vi "Pop-up New Error Window.vi"(8 "Error In":errorcluster, 10 "Error Message":string, 11 "Error Code":i32) -> (0 "Error Out":errorcluster)   [LabVIEW 2023, in "Error Manager.lvlib"]
doc: "Enqueues a message (a command)"
uses:
  Error Manager.lvlib
  Queues/New Error Window Loop Queue/Command (enum).ctl
  Error Display Window/Error Details (cluster).ctl
  Queues/New Error Window Loop Queue/New Error Window Loop Queue.lvclass
  Error Display Window/Error Display Window.lvclass
panel:
  # "Development\ncontrols/indicators useful for development and testing, but which are not outputs of the VI"
  # "Input\nInputs to the VI"
  # "Output\nOutputs of the VI"
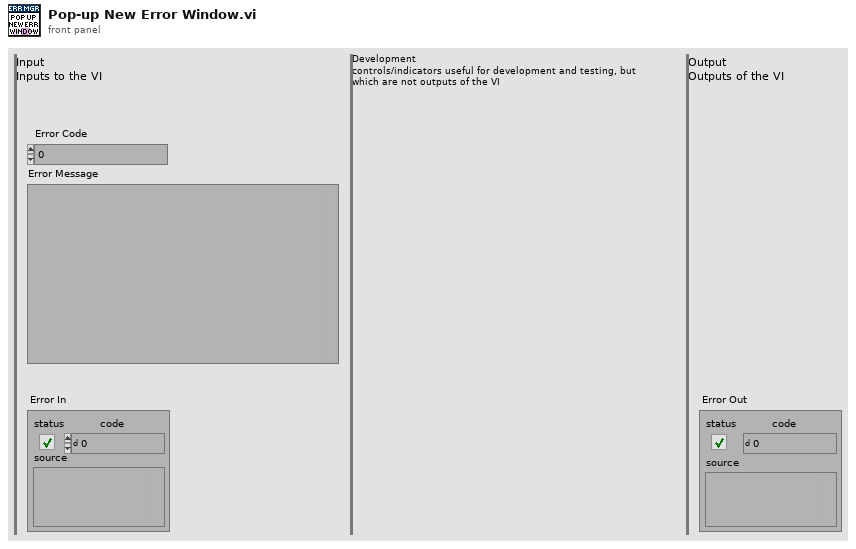
[diagram p1: front panel]
types:
  T1 = typedef "Error Manager.lvlib/New Error Window Loop Queue.lvclass/Command (enum).ctl" = enum16{"Init Loop", "Close Loop", "Pop-up New Error Dialogue"}
  T2 = typedef "Error Manager.lvlib/Error Display Window.lvclass/Error Details (cluster).ctl" = cluster{"Error Code":i32, "Error Message":string}
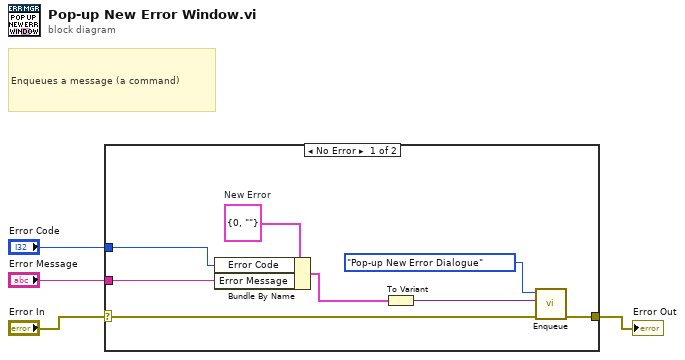
[diagram p0: block diagram]
diagram:
  # "Enqueues a message (a command)"
  n1 = case shown="No Error" "Error In" {
    selector: "Error In" -> [w12 w13]
    tunnel: [w11 w13] -> w3
    tunnel: "Error Code" -> [w6 _]
    tunnel: "Error Message" -> [w5 _]
    frame No Error {
      w8 = T2 {"Error Code"=0, "Error Message"=""}  # New Error
      n2 = Bundle By Name(cluster=w8, "Error Code"=w6, "Error Message"=w5) -> (w7:T2)
      n3 = To Variant(anything=w7) -> (Variant=w9:variant)
      n4 = call "Enqueue.vi"("error in (no error)"=w12, "Data"=w9, "Command"=Command_(enum)."Pop-up New Error Dialogue") -> ("error out"=w11:errorcluster)  [unwired: 8 in]
    }
    frame Error {
    }
  }
  "Error Out" <- w3
